vi "Address to Parity.vi"(8 "String_B":bool, 9 "Address":u16 format="%x") -> (0 "Odd Parity":bool, 1 "Even Parity":bool)   [LabVIEW 2019]
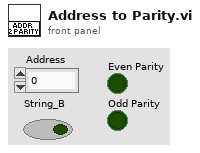
[diagram p1: front panel]
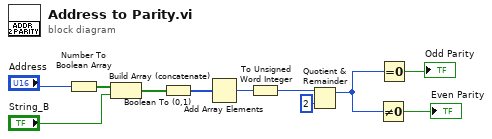
[diagram p0: block diagram]
diagram:
  n1 = Number To Boolean Array(number="Address") -> (Boolean array=w10:bool[])
  n2 = Build Array (concatenate)(w10, "String_B") -> (w2:bool[])
  n3 = Boolean To (0,1)(Boolean=w2) -> (0, 1=w9:i16[])
  n4 = Add Array Elements(numeric array=w9) -> (sum=w7:i16)
  n5 = To Unsigned Word Integer(number=w7) -> (unsigned 16bit integer=w6:u16)
  n6 = Quotient & Remainder(x=w6, y=u16 2) -> (x-y*floor(x/y)=w5:u16)  [unwired: 1 out]
  n7 = Not Equal To 0?(x=w5) -> (x != 0?=→"Even Parity":bool)
  n8 = Equal To 0?(x=w5) -> (x = 0?=→"Odd Parity":bool)
